vi "Load and Vin SMU Measurement.vi"() -> ()   [LabVIEW 2021]
doc: "Demonstrates how to use the DC Voltage Output Function to force an output voltage. This example initializes a session, configures the Output Function, Sense, Autorange, Voltage Level and Current Limit, initiates generation, waits for a specified delay, and measures the voltage and current output. This example uses Single Point source mode."
uses:
  <instrlib>/niDMM/nidmm.llb/niDMM Resolution in Digits.ctl
  <instrlib>/niDMM/nidmm.llb/niDMM Function.ctl
  <instrlib>/niDCPower/nidcpower.llb/niDCPower Output Function.ctl
  <instrlib>/niDCPower/nidcpower.llb/niDCPower Source Mode.ctl
  <instrlib>/niDMM/nidmm.llb/niDMM Configure Measurement Digits.vi
panel:
  out "SMU Measurement":dbl format="%.6p"
  in  "SMU DMM":refnum<k15>="Dev1"
  in  "SMU DMM Measurement":T1
  out "SMU DMM Resolution":dbl caption="SMU Absolute Resolution" format="%#_3p"
  in  "SMU Resolution in Digits":T2=5.5 items=["3 1/2"=3.5, "4 1/2"=4.5, "5 1/2"=5.5, "6 1/2"=6.5, "7 1/2"=7.5]
  out "Load Voltage":dbl caption="SMU Measurement" format="%.6p"
  in  "SMU Range":dbl=10.0 format="%.2f"
  in  "Load DMM":refnum<k15>="Dev1"
  in  "Load DMM Measurement":T1 caption="SMU DMM Measurement"
  out "Load DMM Measurement":dbl caption="SMU Absolute Resolution" format="%#_3p"
  in  "Load DMM Resolution":T2=5.5 caption="SMU Resolution in Digits" items=["3 1/2"=3.5, "4 1/2"=4.5, "5 1/2"=5.5, "6 1/2"=6.5, "7 1/2"=7.5]
  in  "Load SMU":refnum<k15>="Dev1"
  in  "Load SMU Channel":string="0"
  out "Load SMU Current":dbl
  out "Load SMU Voltage":dbl
  in  "error in":errorcluster
  out "error out":errorcluster
  out "Voltage Measurement":dbl caption="Vin SMU Voltage"
  out "Current Measurement":dbl caption="Vin SMU Current"
  in  "Current Limit":dbl=0.01 format="%.3p"
  in  "Voltage Level":dbl=2.0 format="%.5p"
  in  "Vin SMU Channel":string="0"
  in  "Vin SMU":refnum<k15>="Dev1"
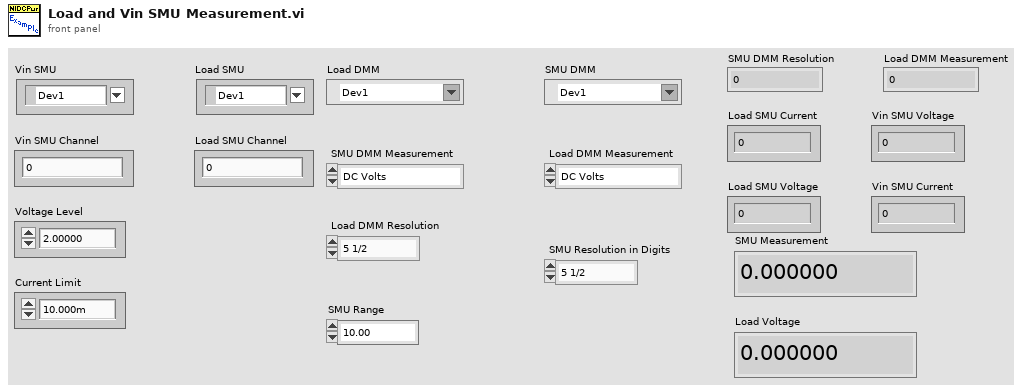
[diagram p1: front panel]
types:
  T1 = typedef "niDMM Function.ctl" = enum16{"DC Volts", "AC Volts", "DC Current", "AC Current", "2-wire Resistance", "4-wire Resistance", "Diode", "Frequency", "Period", "AC Volts DC Coupled", "Capacitance", "Inductance", "Temperature"}
  T2 = typedef "niDMM Resolution in Digits.ctl" = dbl
  T3 = typedef "niDCPower Output Function.ctl" = i32
  T4 = typedef "niDCPower Source Mode.ctl" = i32
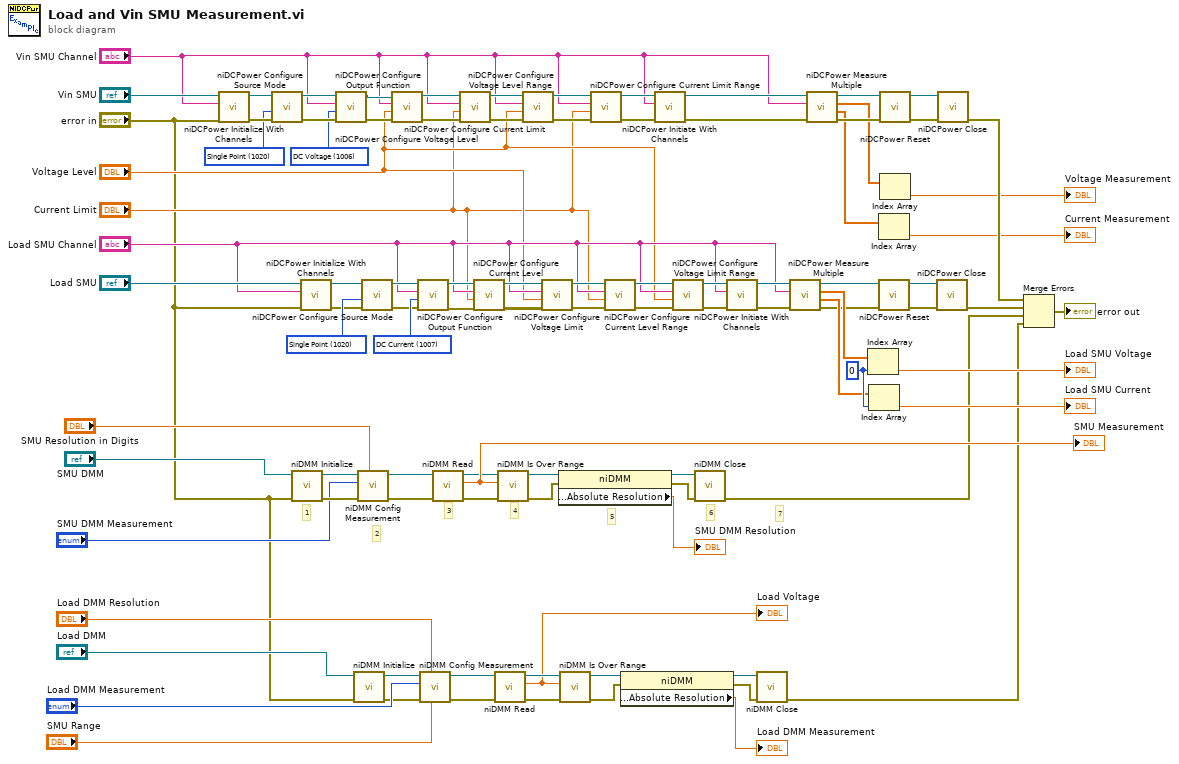
[diagram p0: block diagram]
diagram:
  w68 = T3 1007 items=["DC Voltage"=1006, "DC Current"=1007, "Pulse Voltage"=1049, "Pulse Current"=1050] ("output function")
  w59 = 0 ("index")
  w50 = T4 1020 items=["Single Point"=1020, "Sequence"=1021] ("source mode")
  w74 = T3 1006 items=["DC Voltage"=1006, "DC Current"=1007, "Pulse Voltage"=1049, "Pulse Current"=1050] ("output function")
  w87 = T4 1020 items=["Single Point"=1020, "Sequence"=1021] ("source mode")
  # "2"
  # "1"
  # "7"
  # "6"
  # "5"
  # "4"
  # "3"
  n1 = call <instrlib>:"niDCPower Initialize With Channels.vi"("error in (no error)"="error in", "channels"="Vin SMU Channel", "resource name"="Vin SMU") -> ("error out"=w91:errorcluster, "instrument handle out"=w90:refnum<k15>)  [unwired: 2 in, 5 out]
  n2 = call <instrlib>:"niDCPower Configure Source Mode.vi"("error in (no error)"=w91, "source mode"=w87, "instrument handle"=w90) -> ("error out"=w89:errorcluster, "instrument handle out"=w88:refnum<k15>)  [unwired: 7 out]
  n3 = call <instrlib>:"niDMM Initialize.vi"("error in (no error)"="error in", "Instrument Descriptor"="SMU DMM") -> ("error out"=w11:errorcluster, "instrument handle out"=w12:refnum<k15>)  [unwired: 8 in]
  n4 = call <instrlib>:"niDCPower Initialize With Channels.vi"("error in (no error)"="error in", "channels"="Load SMU Channel", "resource name"="Load SMU") -> ("error out"=w46:errorcluster, "instrument handle out"=w47:refnum<k15>)  [unwired: 2 in, 5 out]
  n5 = call <instrlib>:"niDCPower Configure Output Function.vi"("error in (no error)"=w89, "output function"=w74, "channel name"="Vin SMU Channel", "instrument handle"=w88) -> ("error out"=w75:errorcluster, "instrument handle out"=w76:refnum<k15>)  [unwired: 6 out]
  n6 = call <instrlib>:"niDMM Initialize.vi"("error in (no error)"="error in", "Instrument Descriptor"="Load DMM") -> ("error out"=w26:errorcluster, "instrument handle out"=w25:refnum<k15>)  [unwired: 8 in]
  n7 = call-poly <instrlib>:"niDMM Config Measurement.vi"("Resolution in Digits"="SMU Resolution in Digits", "error in (no error)"=w11, "Function"="SMU DMM Measurement", "instrument handle"=w12) -> ("error out"=w5:errorcluster, "instrument handle out"=w6:refnum<k15>)  [unwired: 6 in]
  n8 = call <instrlib>:"niDCPower Configure Source Mode.vi"("error in (no error)"=w46, "source mode"=w50, "instrument handle"=w47) -> ("error out"=w48:errorcluster, "instrument handle out"=w49:refnum<k15>)  [unwired: 7 out]
  n9 = call <instrlib>:"niDCPower Configure Voltage Level.vi"("error in (no error)"=w75, "voltage level"="Voltage Level", "channel name"="Vin SMU Channel", "instrument handle"=w76) -> ("error out"=w94:errorcluster, "instrument handle out"=w95:refnum<k15>)  [unwired: 6 out]
  n10 = call <instrlib>:"niDCPower Configure Output Function.vi"("error in (no error)"=w48, "output function"=w68, "channel name"="Load SMU Channel", "instrument handle"=w49) -> ("error out"=w66:errorcluster, "instrument handle out"=w67:refnum<k15>)  [unwired: 6 out]
  n11 = call-poly <instrlib>:"niDMM Config Measurement.vi"("Range"="SMU Range", "Resolution in Digits"="Load DMM Resolution", "error in (no error)"=w26, "Function"="Load DMM Measurement", "instrument handle"=w25) -> ("error out"=w32:errorcluster, "instrument handle out"=w31:refnum<k15>)  [unwired: 5 in]
  n12 = call <instrlib>:"niDMM Read.vi"("error in (no error)"=w5, "instrument handle"=w6) -> ("error out"=w8:errorcluster, "Measurement"=w9:dbl, "instrument handle out"=w7:refnum<k15>)  [unwired: 7 in]
  "SMU Measurement" <- w9
  n13 = call <instrlib>:"niDCPower Configure Current Limit.vi"("error in (no error)"=w94, "current limit"="Current Limit", "channel name"="Vin SMU Channel", "instrument handle"=w95) -> ("error out"=w86:errorcluster, "instrument handle out"=w85:refnum<k15>)  [unwired: 1 in, 5 out]
  n14 = call <instrlib>:"niDCPower Configure Current Level.vi"("error in (no error)"=w66, "current level"="Current Limit", "channel name"="Load SMU Channel", "instrument handle"=w67) -> ("error out"=w43:errorcluster, "instrument handle out"=w42:refnum<k15>)  [unwired: 6 out]
  n15 = call <instrlib>:"niDMM Read.vi"("error in (no error)"=w32, "instrument handle"=w31) -> ("error out"=w29:errorcluster, "Measurement"=w28:dbl, "instrument handle out"=w30:refnum<k15>)  [unwired: 7 in]
  "Load Voltage" <- w28
  n16 = call <instrlib>:"niDMM Is Over Range.vi"("error in (no error)"=w8, "Measurement"=w9, "instrument handle"=w7) -> ("error out"=w15:errorcluster, "instrument handle out"=w13:refnum<k15>)  [unwired: 6 in, 1 out]
  n17 = call <instrlib>:"niDCPower Configure Voltage Level Range.vi"("error in (no error)"=w86, "voltage level range"="Voltage Level", "channel name"="Vin SMU Channel", "instrument handle"=w85) -> ("error out"=w84:errorcluster, "instrument handle out"=w83:refnum<k15>)  [unwired: 6 out]
  n18 = call <instrlib>:"niDCPower Configure Voltage Limit.vi"("error in (no error)"=w43, "voltage limit"="Voltage Level", "channel name"="Load SMU Channel", "instrument handle"=w42) -> ("error out"=w51:errorcluster, "instrument handle out"=w52:refnum<k15>)  [unwired: 6 out]
  n19 = property class="niDMM"(reference=w13, error in=w15) -> (reference out=w14:refnum<k15>, error out=w16:errorcluster, "Configuration:Absolute Resolution"=→"SMU DMM Resolution":dbl)
  n20 = call <instrlib>:"niDMM Is Over Range.vi"("error in (no error)"=w29, "Measurement"=w28, "instrument handle"=w30) -> ("error out"=w22:errorcluster, "instrument handle out"=w24:refnum<k15>)  [unwired: 6 in, 1 out]
  n21 = call <instrlib>:"niDCPower Configure Current Limit Range.vi"("error in (no error)"=w84, "current limit range"="Current Limit", "channel name"="Vin SMU Channel", "instrument handle"=w83) -> ("error out"=w79:errorcluster, "instrument handle out"=w80:refnum<k15>)  [unwired: 6 out]
  n22 = call <instrlib>:"niDCPower Configure Current Level Range.vi"("error in (no error)"=w51, "current level range"="Current Limit", "channel name"="Load SMU Channel", "instrument handle"=w52) -> ("error out"=w53:errorcluster, "instrument handle out"=w54:refnum<k15>)  [unwired: 6 out]
  n23 = property class="niDMM"(reference=w24, error in=w22) -> (reference out=w23:refnum<k15>, error out=w21:errorcluster, "Configuration:Absolute Resolution"=→"Load DMM Measurement":dbl)
  n24 = call <instrlib>:"niDCPower Initiate With Channels.vi"("error in (no error)"=w79, "channel name"="Vin SMU Channel", "instrument handle"=w80) -> ("error out"=w77:errorcluster, "instrument handle out"=w78:refnum<k15>)  [unwired: 7 in]
  n25 = call <instrlib>:"niDCPower Configure Voltage Limit Range.vi"("error in (no error)"=w53, "voltage limit range"="Voltage Level", "channel name"="Load SMU Channel", "instrument handle"=w54) -> ("error out"=w63:errorcluster, "instrument handle out"=w62:refnum<k15>)  [unwired: 6 out]
  n26 = call <instrlib>:"niDMM Close.vi"("error in (no error)"=w16, "instrument handle"=w14) -> ("error out"=w2:errorcluster)  [unwired: 9 in]
  n27 = call <instrlib>:"niDCPower Initiate With Channels.vi"("error in (no error)"=w63, "channel name"="Load SMU Channel", "instrument handle"=w62) -> ("error out"=w65:errorcluster, "instrument handle out"=w64:refnum<k15>)  [unwired: 7 in]
  n28 = call <instrlib>:"niDMM Close.vi"("error in (no error)"=w21, "instrument handle"=w23) -> ("error out"=w1:errorcluster)  [unwired: 9 in]
  n29 = call <instrlib>:"niDCPower Measure Multiple.vi"("error in (no error)"=w65, "channel name"="Load SMU Channel", "instrument handle"=w64) -> ("error out"=w56:errorcluster, "current measurements"=w58:dbl[], "voltage measurements"=w57:dbl[], "instrument handle out"=w55:refnum<k15>)  [unwired: 5 out]
  n30 = call <instrlib>:"niDCPower Measure Multiple.vi"("error in (no error)"=w77, "channel name"="Vin SMU Channel", "instrument handle"=w78) -> ("error out"=w81:errorcluster, "current measurements"=w72:dbl[], "voltage measurements"=w70:dbl[], "instrument handle out"=w82:refnum<k15>)  [unwired: 5 out]
  n31 = Index Array(array=w57, index=w59) -> (element=→"Load SMU Voltage":dbl)
  n32 = Index Array(array=w58, index=w59) -> (element=→"Load SMU Current":dbl)
  n33 = Index Array(array=w72) -> (element=→"Current Measurement":dbl)  [unwired: 1 in]
  n34 = call <instrlib>:"niDCPower Reset.vi"("error in (no error)"=w56, "instrument handle"=w55) -> ("error out"=w45:errorcluster, "instrument handle out"=w44:refnum<k15>)  [unwired: 2 in, 6 out]
  n35 = call <instrlib>:"niDCPower Reset.vi"("error in (no error)"=w81, "instrument handle"=w82) -> ("error out"=w92:errorcluster, "instrument handle out"=w93:refnum<k15>)  [unwired: 2 in, 6 out]
  n36 = Index Array(array=w70) -> (element=→"Voltage Measurement":dbl)  [unwired: 1 in]
  n37 = call <instrlib>:"niDCPower Close.vi"("error in (no error)"=w45, "instrument handle"=w44) -> ("error out"=w39:errorcluster)  [unwired: 9 out]
  n38 = call <instrlib>:"niDCPower Close.vi"("error in (no error)"=w92, "instrument handle"=w93) -> ("error out"=w73:errorcluster)  [unwired: 9 out]
  n39 = Merge Errors(w73, w39, w2, w1) -> (→"error out":errorcluster)
